vi "02AMT800_RPMmeasure.vi"() -> ()   [LabVIEW 2017]
uses:
  <vilib>/Analysis/baseanly.llb/Mean (DBL).vi
  <vilib>/Utility/file.llb/Write Delimited Spreadsheet (DBL).vi
  <vilib>/Analysis/NI_AALBase.lvlib
panel:
  out "TIME":dbl format="%<%H:%M:%S>t"
  out "XY Graph":cluster{dbl[], dbl[]}(graph)
  out "SPM":dbl format="%0.2f"
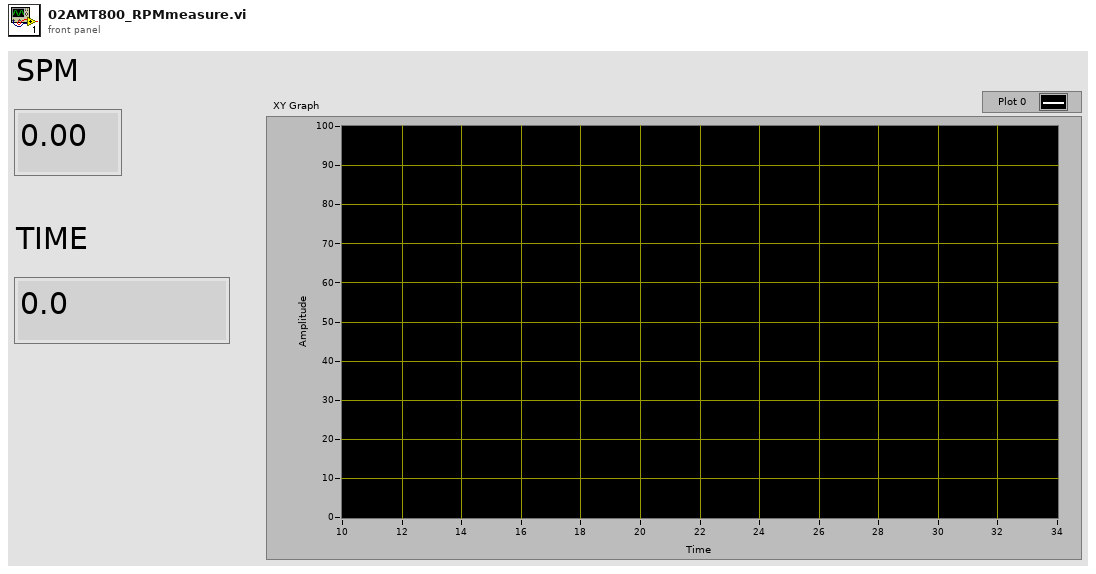
[diagram p1: front panel]
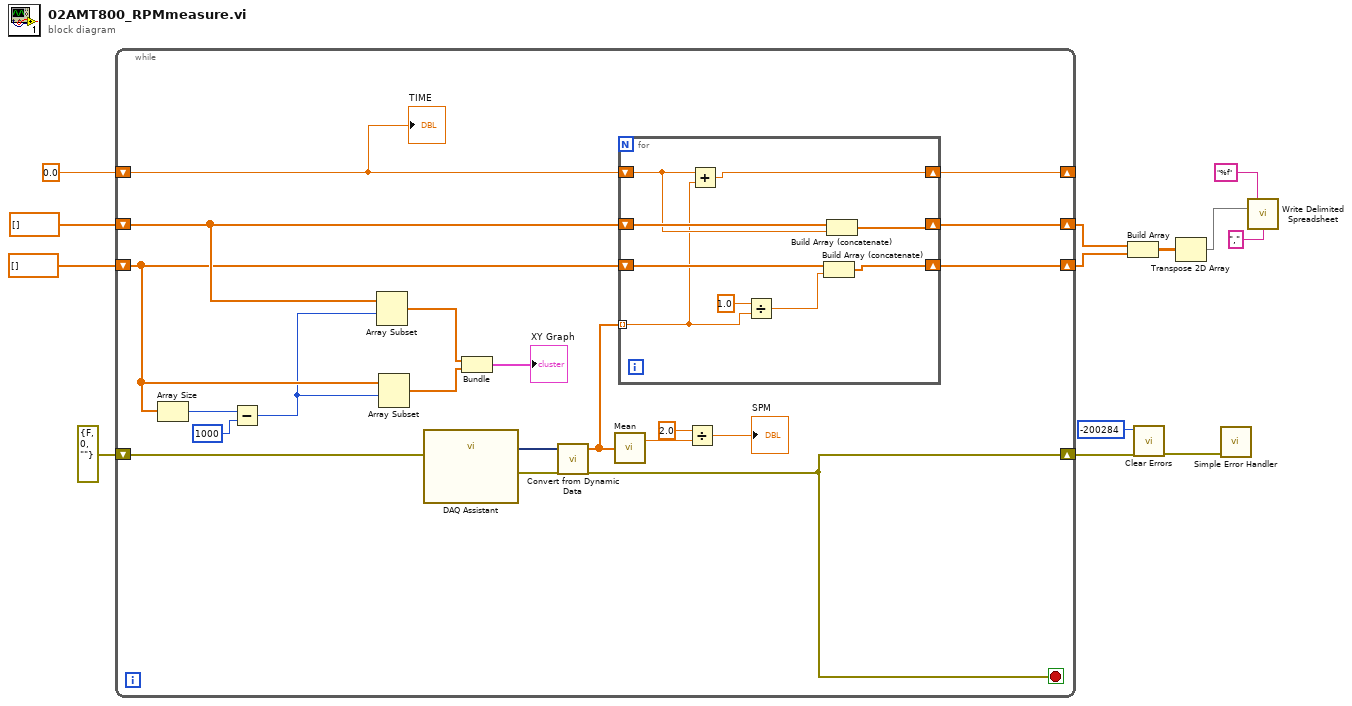
[diagram p0: block diagram]
diagram:
  n1 = while {
    shift-right: [w27] -> w9
    shift-left: errorcluster {"status"=FALSE, "code"=0, "source"=""} ("error out") -> [w32]
    shift-right: [w24] -> w6
    shift-left: dbl[] [] -> [w20]
    shift-right: [w25] -> _
    shift-left: 0.0 -> [w21]
    shift-right: [w23] -> w5
    shift-left: dbl[] [] -> [w17]
    stop <- w27 stop-if-true
    n2 = Array Size(array=w17) -> (size(s)=w16:i32)
    n3 = Subtract(x=w16, y=1000) -> (x-y=w14:i32)
    n4 = Array Subset(array=w20, index=w14) -> (w18:dbl[])  [unwired: 1 in]
    n5 = Array Subset(array=w17, index=w14) -> (w19:dbl[])  [unwired: 1 in]
    n6 = call "DAQ Assistant"("error in"=w32) -> ("data"=w31:dynamicdata, "error out"=w27:errorcluster)  [unwired: 15 in, 2 out]
    n7 = Bundle(w18, w19) -> (→"XY Graph":cluster{dbl[], dbl[]})  [unwired: 1 in]
    n8 = call "Convert from Dynamic Data"("Dynamic Data Type"=w31) -> ("Array"=w26:dbl[])  [unwired: 3 in]
    n9 = call-poly <vilib>:"Mean.vi"("X"=w26) -> ("mean"=w30:dbl)  [unwired: 1 out]
    n10 = for {
      tunnel: w26 -> [w35] mode=indexing
      shift-right: [w39] -> w24
      shift-left: w20 -> [w40]
      shift-right: [w41] -> w25
      shift-left: w21 -> [w38]
      shift-right: [w33] -> w23
      shift-left: w17 -> [w37]
      n11 = Add(x=w38, y=w35) -> (x+y=w41:dbl)
      n12 = Divide(x=1.0, y=w35) -> (x/y=w34:dbl)
      n13 = Build Array (concatenate)(w37, w34) -> (w33:dbl[])
      n14 = Build Array (concatenate)(w40, w38) -> (w39:dbl[])
    }
    n15 = Divide(x=2.0, y=w30) -> (x/y=→"SPM":dbl)
    "TIME" <- w21
  }
  n16 = Build Array(w6, w5) -> (w3:dbl[][])
  n17 = call <vilib>:"Clear Errors.vi"("error in (no error)"=w9, "specific error code to clear (0: all)"=-200284) -> ("error out"=w8:errorcluster)  [unwired: 4 in, 1 out]
  n18 = Transpose 2D Array(2D array=w3) -> (transposed array=w2:dbl[][])
  n19 = call <vilib>:"Simple Error Handler.vi"("error in (no error)"=w8) -> ()  [unwired: 4 in, 5 out]
  n20 = call-poly <vilib>:"Write Delimited Spreadsheet.vi"("format (%.3f)"="%f", "2D data"=w2, "delimiter (\\t)"="," ("delimiter (\\t)")) -> ()  [unwired: 11 in, 2 out]
